vi "BrkPtPRF.vi"(2 "error in":errorcluster, 3 "PRF (1 ms)":u32=1 min=1 max=2147483647, 4 "Bd ID in":u8=1) -> (0 "error out":errorcluster, 1 "Bd ID Out":u8=1)   [LabVIEW 2022 SP3]
uses:
  <vilib>/Motion/FlexMotion/FunctionsVIs/MotionIO.llb/Set Breakpoint Output MOMO (8 axes).flx
  <vilib>/Motion/FlexMotion/CustomControls/CustomControls.llb/Mask (8 axes).flx
  <vilib>/Motion/FlexMotion/FunctionsVIs/OnboardProgramming.llb/Jump to Label on Condition (8 axes).flx
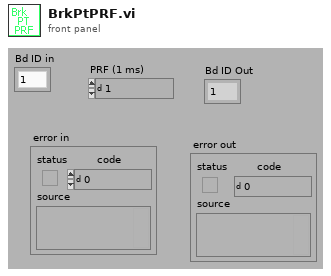
[diagram p1: front panel]
types:
  T1 = typedef "Mask (8 axes).flx" = cluster{"1":bool, "2":bool, "3":bool, "4":bool, "5":bool, "6":bool, "7":bool, "8":bool}
  T2 = typedef "Bd Id Out" = u8
  T3 = typedef "Resource Out.flx" = u8
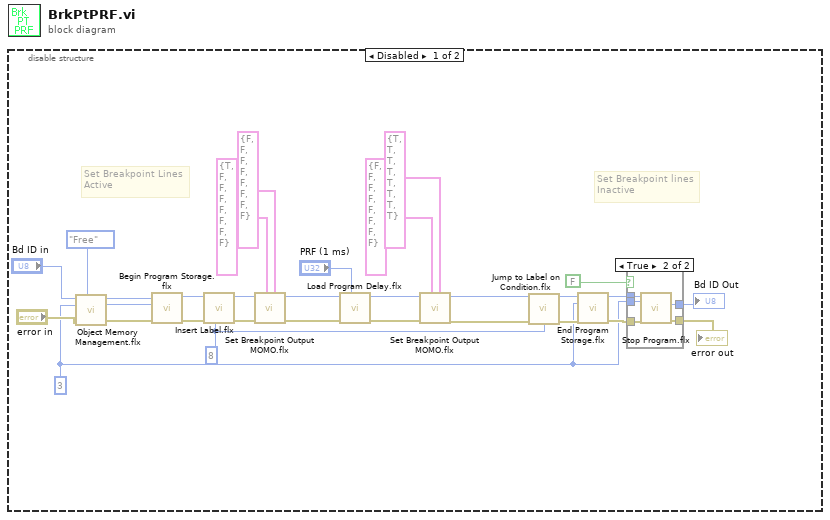
[diagram p0: block diagram]
diagram:
  n1 = disable-structure shown="Disabled" {
    frame Disabled {
      w22 = 8
      w12 = 3
      # "Set Breakpoint Lines\nActive"
      # "Set Breakpoint lines\nInactive"
      n2 = call <vilib>:"Object Memory Management.flx"("Operation"=enum16{"Save", "Delete", "Free"}."Free", "error in (no error)"="error in", "Object (1)"=w12, "Board ID"="Bd ID in") -> ("error out"=w15:errorcluster, "Bd ID Out"=w16:T2)  [unwired: 4 out]
      n3 = call <vilib>:"Begin Program Storage.flx"("error in (no error)"=w15, "Program (1)"=w12, "Board ID"=w16) -> ("error out"=w28:errorcluster, "Bd ID Out"=w29:T2)  [unwired: 4 out]
      n4 = call <vilib>:"Insert Label.flx"("Label Number (1)"=w22, "error in (no error)"=w28, "Board ID"=w29) -> ("error out"=w26:errorcluster, "Bd ID Out"=w27:T2)  [unwired: 4 out]
      n5 = call-poly <vilib>:"Set Breakpoint Output MOMO.flx"("Must Off (False)"=T1 {"1"=FALSE, "2"=FALSE, "3"=FALSE, "4"=FALSE, "5"=FALSE, "6"=FALSE, "7"=FALSE, "8"=FALSE}, "Must On (False)"=T1 {"1"=TRUE, "2"=FALSE, "3"=FALSE, "4"=FALSE, "5"=FALSE, "6"=FALSE, "7"=FALSE, "8"=FALSE}, "error in (no error)"=w26, "Board ID"=w27) -> ("error out"=w9:errorcluster, "Bd ID Out"=w10:T2)  [unwired: 2 in, 2 out]
      n6 = call <vilib>:"Load Program Delay.flx"("Delay Value (1 ms)"="PRF (1 ms)", "error in (no error)"=w9, "Board ID"=w10) -> ("error out"=w7:errorcluster, "Bd ID Out"=w8:T2)  [unwired: 4 out]
      n7 = call-poly <vilib>:"Set Breakpoint Output MOMO.flx"("Must Off (False)"=T1 {"1"=TRUE, "2"=TRUE, "3"=TRUE, "4"=TRUE, "5"=TRUE, "6"=TRUE, "7"=TRUE, "8"=TRUE}, "Must On (False)"=T1 {"1"=FALSE, "2"=FALSE, "3"=FALSE, "4"=FALSE, "5"=FALSE, "6"=FALSE, "7"=FALSE, "8"=FALSE}, "error in (no error)"=w7, "Board ID"=w8) -> ("error out"=w5:errorcluster, "Bd ID Out"=w6:T2)  [unwired: 2 in, 2 out]
      n8 = call-poly <vilib>:"Jump to Label on Condition.flx"("Board ID"=w6, "error in (no error)"=w5, "Jump to Label (1)"=w22) -> ("Bd ID Out"=w24:T2, "error out"=w23:errorcluster)  [unwired: 5 in, 6 out]
      n9 = call <vilib>:"End Program Storage.flx"("error in (no error)"=w23, "Program (1)"=w12, "Board ID"=w24) -> ("error out"=w19:errorcluster, "Bd ID Out"=w20:T2)  [unwired: 4 out]
      n10 = case shown="True" FALSE ("Case Constant\n(See Context Help)") {
        tunnel: [w31 w36] -> w21
        tunnel: w20 -> [w31 w35]
        tunnel: w19 -> [w30 w34]
        tunnel: w12 -> [_ w33]
        tunnel: [w30 w32] -> w18
        frame False {
        }
        frame True {
          n11 = call <vilib>:"Stop Program.flx"("error in (no error)"=w34, "Program (1)"=w33, "Board ID"=w35) -> ("error out"=w32:errorcluster, "Resource Out"=w36:T3)  [unwired: 1 in, 3 out]
        }
      }
      "error out" <- w18
      "Bd ID Out" <- w21
    }
    frame Enabled {
    }
  }
